vi "apply_matrix_transformation_to_spots.vi"(4 "Transform centre (i.e. transform about this point)":cluster{"x":dbl, "y":dbl, "z":dbl}, 5 "Transformation Matrix (3x3)":T3, 8 "Spot In":T1 {"Amplitude Correction" step=0.1; "Line Trapping"."Phase Gradient" step=0.05; "Line Trapping"."Vector"."x" step=1e-06 format="%#_6p"; "Line Trapping"."Vector"."y" step=1e-06 format="%#_6p"; "Line Trapping"."Vector"."z" step=1e-06 format="%#_6p"; "NA Position"."r" step=1e-06; "NA Position"."y" step=1e-06; "NA Position"."x" step=1e-06; "Position"."z" step=1e-06; "Position"."y" step=1e-06; "Position"."x" step=1e-06; "Phase" step=0.7753; "Intensity" step=0.1}) -> (3 "Spot Out":T1 {"Amplitude Correction" step=0.1; "Line Trapping"."Phase Gradient" step=0.05; "Line Trapping"."Vector"."x" step=1e-06 format="%#_6p"; "Line Trapping"."Vector"."y" step=1e-06 format="%#_6p"; "Line Trapping"."Vector"."z" step=1e-06 format="%#_6p"; "NA Position"."r" step=1e-06; "NA Position"."y" step=1e-06; "NA Position"."x" step=1e-06; "Position"."z" step=1e-06; "Position"."y" step=1e-06; "Position"."x" step=1e-06; "Phase" step=0.7753; "Intensity" step=0.1})   [LabVIEW 2010]
uses:
  <vilib>/Analysis/Matrix/Datatypes/RealMatrix.ctl
  spot.ctl
  line_trapping.ctl
  <vilib>/Analysis/Matrix/NI_Matrix.lvlib
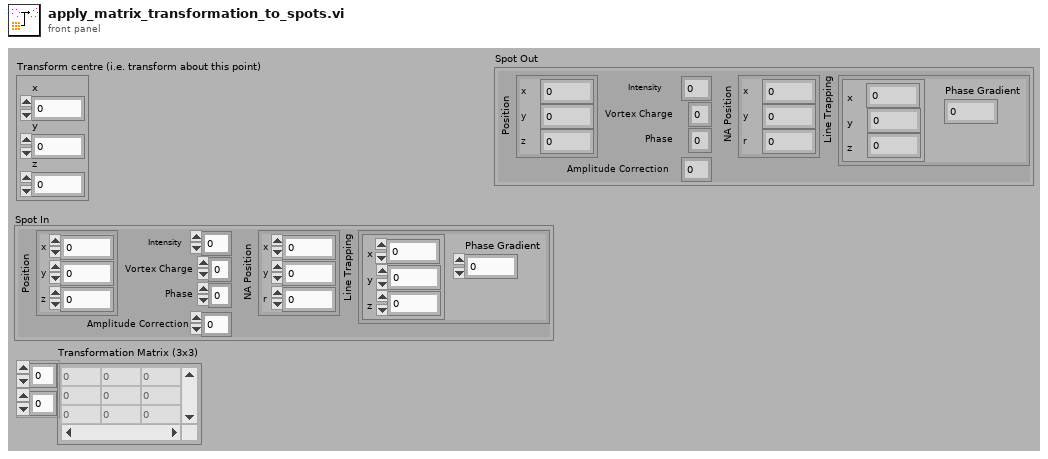
[diagram p1: front panel]
types:
  T1 = typedef "spot.ctl" = cluster{"Position":cluster{"x":dbl, "y":dbl, "z":dbl}, "Intensity":dbl, "Vortex Charge":i8, "Phase":dbl, "NA Position":cluster{"x":dbl, "y":dbl, "r":dbl}, "Line Trapping":T2, "Amplitude Correction":dbl}
  T2 = typedef "line_trapping.ctl" = cluster{"Vector":cluster{"x":dbl, "y":dbl, "z":dbl}, "Phase Gradient":dbl}
  T3 = typedef "NI_Matrix.lvlib/RealMatrix.ctl" = dbl[][]
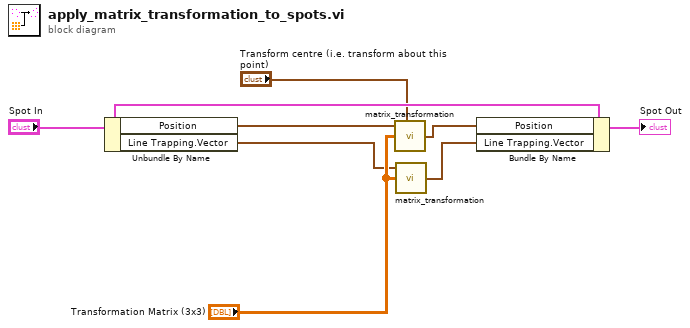
[diagram p0: block diagram]
diagram:
  n1 = Unbundle By Name("Spot In") -> ("Position"=w2:cluster{"x":dbl, "y":dbl, "z":dbl}, "Line Trapping.Vector"=w6:cluster{"x":dbl, "y":dbl, "z":dbl})
  n2 = call "matrix_transformation.vi"("Transformation Centre"="Transform centre (i.e. transform about this point)", "Transformation Matrix"="Transformation Matrix (3x3)", "Input Vector"=w2) -> ("Output Vector"=w5:cluster{dbl, dbl, dbl})  [unwired: 1 out]
  n3 = call "matrix_transformation.vi"("Transformation Matrix"="Transformation Matrix (3x3)", "Input Vector"=w6) -> ("Output Vector"=w8:cluster{dbl, dbl, dbl})  [unwired: 1 in, 1 out]
  n4 = Bundle By Name(cluster="Spot In", "Position"=w5, "Line Trapping.Vector"=w8) -> (→"Spot Out":T1)
